vi "Joystick_Normalize.vi"(7 "Power":sgl=100.0, 11 "Joystick In":i8) -> (3 "Norm Out":sgl)   [LabVIEW 2012, in "Serenity_mk2.lvrbt"]
doc: "converts joystick input to motor power."
uses:
  Serenity_mk2.lvrbt
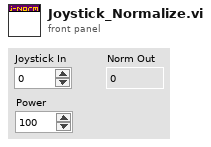
[diagram p1: front panel]
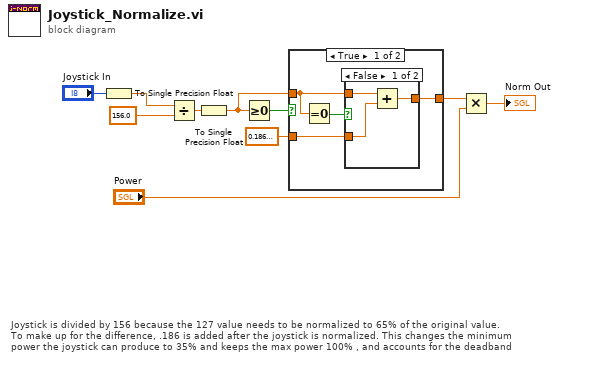
[diagram p0: block diagram]
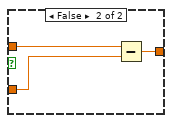
[diagram p3: hidden frame]
diagram:
  # "Joystick is divided by 156 because the 127 value needs to be normalized to 65% of the original value.\nTo make up for the difference, .186 is added after the joystick is normalized. This changes the minimum\npower the joystick can produce to 35% and keeps the max power 100% , and accounts for the deadband"
  n1 = To Single Precision Float(number="Joystick In") -> (single precision float=w5:sgl)
  n2 = Divide(x=w5, y=sgl 156.0) -> (x/y=w8:sgl)
  n3 = To Single Precision Float(number=w8) -> (single precision float=w3:sgl)
  n4 = Greater Or Equal To 0?(x=w3) -> (x >= 0?=w4:bool)
  n5 = case shown="True" w4 {
    tunnel: w3 -> [w12 w21]
    tunnel: sgl 0.186 ("y") -> [w11 w20]
    tunnel: [w14 w19] -> w1
    frame True {
      n6 = Equal To 0?(x=w12) -> (x = 0?=w13:bool)
      n7 = case shown="False" w13 {
        tunnel: w12 -> [w17 w18]
        tunnel: w11 -> [w16 _]
        tunnel: [w15 w18] -> w14
        frame False {
          n8 = Add(x=w17, y=w16) -> (x+y=w15:sgl)
        }
        frame True {
        }
      }
    }
    frame False {
      n9 = Subtract(x=w21, y=w20) -> (x-y=w19:sgl)
    }
  }
  n10 = Multiply(x=w1, y="Power") -> (x*y=→"Norm Out":sgl)
